vi "SpeedTest.vi"() -> ()   [LabVIEW 2014]
panel:
  out "x/y":dbl
  # "BB  Serial - 50-60 msec per command\nBB - 35 msec per command\nArduino - 20 msec per command"
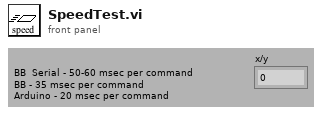
[diagram p1: front panel]
types:
  T1 = typedef "BotSpeak_Control.ctl" = cluster{"Address":string, "Reply EOF":string, "Hardware":string, "Retries":i8, "Timeout":i32, "Open?":bool}
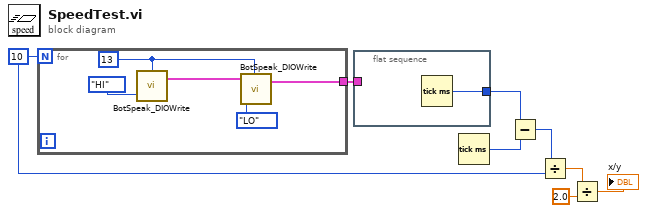
[diagram p0: block diagram]
diagram:
  w6 = 10
  n1 = for {
    N: w6 -> [_]
    tunnel: [w9] -> w5
    w11 = 13
    n2 = call <userlib>:"BotSpeak_DIOWrite.vi"("State"=enum32{"LO", "HI"}."HI", "DIO Line"=w11) -> ("Bot Settings"=w10:T1)  [unwired: 1 in, 1 out]
    n3 = call <userlib>:"BotSpeak_DIOWrite.vi"("State"=enum32{"LO", "HI"}."LO", "Bot Settings"=w10, "DIO Line"=w11) -> ("Bot Settings"=w9:T1)  [unwired: 1 out]
  }
  n4 = flat-sequence {
    tunnel: w5 -> [_]
    tunnel: [w14] -> w4
    frame #0 {
      n5 = Tick Count (ms)() -> (millisecond timer value=w14:u32)
    }
  }
  n6 = Tick Count (ms)() -> (millisecond timer value=w8:u32)
  n7 = Subtract(x=w4, y=w8) -> (x-y=w7:u32)
  n8 = Divide(x=w7, y=w6) -> (x/y=w3:dbl)
  n9 = Divide(x=w3, y=2.0) -> (x/y=→"x/y":dbl)
